vi "FipsAdjacent.vi"() -> (11 "Fips":i32[](array[numeric]))   [LabVIEW 2017] (continued)
County, SC\"\t45075\n\"Edgefield County, SC\"\t45037\t\"Columbia County, GA\"\t13073\n\"Edgefield County, SC\"\t45037\t\"Richmond County, GA\"\t13245\n\"Edgefield County, SC\"\t45037\t\"Aiken County, SC\"\t45003\n\"Edgefield County, SC\"\t45037\t\"Edgefield County, SC\"\t45037\n\"Edgefield County, SC\"\t45037\t\"Greenwood County, SC\"\t45047\n\"Edgefield County, SC\"\t45037\t\"McCormick County, SC\"\t45065\n\"Edgefield County, SC\"\t45037\t\"Saluda County, SC\"\t45081\n\"Fairfield County, SC\"\t45039\t\"Chester County, SC\"\t45023\n\"Fairfield County, SC\"\t45039\t\"Fairfield County, SC\"\t45039\n\"Fairfield County, SC\"\t45039\t\"Kershaw County, SC\"\t45055\n\"Fairfield County, SC\"\t45039\t\"Lancaster County, SC\"\t45057\n\"Fairfield County, SC\"\t45039\t\"Newberry County, SC\"\t45071\n\"Fairfield County, SC\"\t45039\t\"Richland County, SC\"\t45079\n\"Fairfield County, SC\"\t45039\t\"Union County, SC\"\t45087\n\"Florence County, SC\"\t45041\t\"Clarendon County, SC\"\t45027\n\"Florence County, SC\"\t45041\t\"Darlington County, SC\"\t45031\n\"Florence County, SC\"\t45041\t\"Dillon County, SC\"\t45033\n\"Florence County, SC\"\t45041\t\"Florence County, SC\"\t45041\n\"Florence County, SC\"\t45041\t\"Lee County, SC\"\t45061\n\"Florence County, SC\"\t45041\t\"Marion County, SC\"\t45067\n\"Florence County, SC\"\t45041\t\"Marlboro County, SC\"\t45069\n\"Florence County, SC\"\t45041\t\"Sumter County, SC\"\t45085\n\"Florence County, SC\"\t45041\t\"Williamsburg County, SC\"\t45089\n\"Georgetown County, SC\"\t45043\t\"Berkeley County, SC\"\t45015\n\"Georgetown County, SC\"\t45043\t\"Charleston County, SC\"\t45019\n\"Georgetown County, SC\"\t45043\t\"Georgetown County, SC\"\t45043\n\"Georgetown County, SC\"\t45043\t\"Horry County, SC\"\t45051\n\"Georgetown County, SC\"\t45043\t\"Marion County, SC\"\t45067\n\"Georgetown County, SC\"\t45043\t\"Williamsburg County, SC\"\t45089\n\"Greenville County, SC\"\t45045\t\"Henderson County, NC\"\t37089\n\"Greenville County, SC\"\t45045\t\"Polk County, NC\"\t37149\n\"Greenville County, SC\"\t45045\t\"Transylvania County, NC\"\t37175\n\"Greenville County, SC\"\t45045\t\"Abbeville County, SC\"\t45001\n\"Greenville County, SC\"\t45045\t\"Anderson County, SC\"\t45007\n\"Greenville County, SC\"\t45045\t\"Greenville County, SC\"\t45045\n\"Greenville County, SC\"\t45045\t\"Laurens County, SC\"\t45059\n\"Greenville County, SC\"\t45045\t\"Pickens County, SC\"\t45077\n\"Greenville County, SC\"\t45045\t\"Spartanburg County, SC\"\t45083\n\"Greenwood County, SC\"\t45047\t\"Abbeville County, SC\"\t45001\n\"Greenwood County, SC\"\t45047\t\"Edgefield County, SC\"\t45037\n\"Greenwood County, SC\"\t45047\t\"Greenwood County, SC\"\t45047\n\"Greenwood County, SC\"\t45047\t\"Laurens County, SC\"\t45059\n\"Greenwood County, SC\"\t45047\t\"McCormick County, SC\"\t45065\n\"Greenwood County, SC\"\t45047\t\"Newberry County, SC\"\t45071\n\"Greenwood County, SC\"\t45047\t\"Saluda County, SC\"\t45081\n\"Hampton County, SC\"\t45049\t\"Effingham County, GA\"\t13103\n\"Hampton County, SC\"\t45049\t\"Screven County, GA\"\t13251\n\"Hampton County, SC\"\t45049\t\"Allendale County, SC\"\t45005\n\"Hampton County, SC\"\t45049\t\"Bamberg County, SC\"\t45009\n\"Hampton County, SC\"\t45049\t\"Beaufort County, SC\"\t45013\n\"Hampton County, SC\"\t45049\t\"Colleton County, SC\"\t45029\n\"Hampton County, SC\"\t45049\t\"Hampton County, SC\"\t45049\n\"Hampton County, SC\"\t45049\t\"Jasper County, SC\"\t45053\n\"Horry County, SC\"\t45051\t\"Brunswick County, NC\"\t37019\n\"Horry County, SC\"\t45051\t\"Columbus County, NC\"\t37047\n\"Horry County, SC\"\t45051\t\"Robeson County, NC\"\t37155\n\"Horry County, SC\"\t45051\t\"Dillon County, SC\"\t45033\n\"Horry County, SC\"\t45051\t\"Georgetown County, SC\"\t45043\n\"Horry County, SC\"\t45051\t\"Horry County, SC\"\t45051\n\"Horry County, SC\"\t45051\t\"Marion County, SC\"\t45067\n\"Jasper County, SC\"\t45053\t\"Chatham County, GA\"\t13051\n\"Jasper County, SC\"\t45053\t\"Effingham County, GA\"\t13103\n\"Jasper County, SC\"\t45053\t\"Beaufort County, SC\"\t45013\n\"Jasper County, SC\"\t45053\t\"Hampton County, SC\"\t45049\n\"Jasper County, SC\"\t45053\t\"Jasper County, SC\"\t45053\n\"Kershaw County, SC\"\t45055\t\"Chesterfield County, SC\"\t45025\n\"Kershaw County, SC\"\t45055\t\"Darlington County, SC\"\t45031\n\"Kershaw County, SC\"\t45055\t\"Fairfield County, SC\"\t45039\n\"Kershaw County, SC\"\t45055\t\"Kershaw County, SC\"\t45055\n\"Kershaw County, SC\"\t45055\t\"Lancaster County, SC\"\t45057\n\"Kershaw County, SC\"\t45055\t\"Lee County, SC\"\t45061\n\"Kershaw County, SC\"\t45055\t\"Richland County, SC\"\t45079\n\"Kershaw County, SC\"\t45055\t\"Sumter County, SC\"\t45085\n\"Lancaster County, SC\"\t45057\t\"Mecklenburg County, NC\"\t37119\n\"Lancaster County, SC\"\t45057\t\"Union County, NC\"\t37179\n\"Lancaster County, SC\"\t45057\t\"Chester County, SC\"\t45023\n\"Lancaster County, SC\"\t45057\t\"Chesterfield County, SC\"\t45025\n\"Lancaster County, SC\"\t45057\t\"Fairfield County, SC\"\t45039\n\"Lancaster County, SC\"\t45057\t\"Kershaw County, SC\"\t45055\n\"Lancaster County, SC\"\t45057\t\"Lancaster County, SC\"\t45057\n\"Lancaster County, SC\"\t45057\t\"York County, SC\"\t45091\n\"Laurens County, SC\"\t45059\t\"Abbeville County, SC\"\t45001\n\"Laurens County, SC\"\t45059\t\"Anderson County, SC\"\t45007\n\"Laurens County, SC\"\t45059\t\"Greenville County, SC\"\t45045\n\"Laurens County, SC\"\t45059\t\"Greenwood County, SC\"\t45047\n\"Laurens County, SC\"\t45059\t\"Laurens County, SC\"\t45059\n\"Laurens County, SC\"\t45059\t\"Newberry County, SC\"\t45071\n\"Laurens County, SC\"\t45059\t\"Spartanburg County, SC\"\t45083\n\"Laurens County, SC\"\t45059\t\"Union County, SC\"\t45087\n\"Lee County, SC\"\t45061\t\"Darlington County, SC\"\t45031\n\"Lee County, SC\"\t45061\t\"Florence County, SC\"\t45041\n\"Lee County, SC\"\t45061\t\"Kershaw County, SC\"\t45055\n\"Lee County, SC\"\t45061\t\"Lee County, SC\"\t45061\n\"Lee County, SC\"\t45061\t\"Sumter County, SC\"\t45085\n\"Lexington County, SC\"\t45063\t\"Aiken County, SC\"\t45003\n\"Lexington County, SC\"\t45063\t\"Calhoun County, SC\"\t45017\n\"Lexington County, SC\"\t45063\t\"Lexington County, SC\"\t45063\n\"Lexington County, SC\"\t45063\t\"Newberry County, SC\"\t45071\n\"Lexington County, SC\"\t45063\t\"Orangeburg County, SC\"\t45075\n\"Lexington County, SC\"\t45063\t\"Richland County, SC\"\t45079\n\"Lexington County, SC\"\t45063\t\"Saluda County, SC\"\t45081\n\"McCormick County, SC\"\t45065\t\"Columbia County, GA\"\t13073\n\"McCormick County, SC\"\t45065\t\"Elbert County, GA\"\t13105\n\"McCormick County, SC\"\t45065\t\"Lincoln County, GA\"\t13181\n\"McCormick County, SC\"\t45065\t\"Abbeville County, SC\"\t45001\n\"McCormick County, SC\"\t45065\t\"Edgefield County, SC\"\t45037\n\"McCormick County, SC\"\t45065\t\"Greenwood County, SC\"\t45047\n\"McCormick County, SC\"\t45065\t\"McCormick County, SC\"\t45065\n\"Marion County, SC\"\t45067\t\"Dillon County, SC\"\t45033\n\"Marion County, SC\"\t45067\t\"Florence County, SC\"\t45041\n\"Marion County, SC\"\t45067\t\"Georgetown County, SC\"\t45043\n\"Marion County, SC\"\t45067\t\"Horry County, SC\"\t45051\n\"Marion County, SC\"\t45067\t\"Marion County, SC\"\t45067\n\"Marion County, SC\"\t45067\t\"Williamsburg County, SC\"\t45089\n\"Marlboro County, SC\"\t45069\t\"Anson County, NC\"\t37007\n\"Marlboro County, SC\"\t45069\t\"Richmond County, NC\"\t37153\n\"Marlboro County, SC\"\t45069\t\"Robeson County, NC\"\t37155\n\"Marlboro County, SC\"\t45069\t\"Scotland County, NC\"\t37165\n\"Marlboro County, SC\"\t45069\t\"Chesterfield County, SC\"\t45025\n\"Marlboro County, SC\"\t45069\t\"Darlington County, SC\"\t45031\n\"Marlboro County, SC\"\t45069\t\"Dillon County, SC\"\t45033\n\"Marlboro County, SC\"\t45069\t\"Florence County, SC\"\t45041\n\"Marlboro County, SC\"\t45069\t\"Marlboro County, SC\"\t45069\n\"Newberry County, SC\"\t45071\t\"Fairfield County, SC\"\t45039\n\"Newberry County, SC\"\t45071\t\"Greenwood County, SC\"\t45047\n\"Newberry County, SC\"\t45071\t\"Laurens County, SC\"\t45059\n\"Newberry County, SC\"\t45071\t\"Lexington County, SC\"\t45063\n\"Newberry County, SC\"\t45071\t\"Newberry County, SC\"\t45071\n\"Newberry County, SC\"\t45071\t\"Richland County, SC\"\t45079\n\"Newberry County, SC\"\t45071\t\"Saluda County, SC\"\t45081\n\"Newberry County, SC\"\t45071\t\"Union County, SC\"\t45087\n\"Oconee County, SC\"\t45073\t\"Franklin County, GA\"\t13119\n\"Oconee County, SC\"\t45073\t\"Habersham County, GA\"\t13137\n\"Oconee County, SC\"\t45073\t\"Hart County, GA\"\t13147\n\"Oconee County, SC\"\t45073\t\"Rabun County, GA\"\t13241\n\"Oconee County, SC\"\t45073\t\"Stephens County, GA\"\t13257\n\"Oconee County, SC\"\t45073\t\"Jackson County, NC\"\t37099\n\"Oconee County, SC\"\t45073\t\"Macon County, NC\"\t37113\n\"Oconee County, SC\"\t45073\t\"Transylvania County, NC\"\t37175\n\"Oconee County, SC\"\t45073\t\"Anderson County, SC\"\t45007\n\"Oconee County, SC\"\t45073\t\"Oconee County, SC\"\t45073\n\"Oconee County, SC\"\t45073\t\"Pickens County, SC\"\t45077\n\"Orangeburg County, SC\"\t45075\t\"Aiken County, SC\"\t45003\n\"Orangeburg County, SC\"\t45075\t\"Bamberg County, SC\"\t45009\n\"Orangeburg County, SC\"\t45075\t\"Barnwell County, SC\"\t45011\n\"Orangeburg County, SC\"\t45075\t\"Berkeley County, SC\"\t45015\n\"Orangeburg County, SC\"\t45075\t\"Calhoun County, SC\"\t45017\n\"Orangeburg County, SC\"\t45075\t\"Clarendon County, SC\"\t45027\n\"Orangeburg County, SC\"\t45075\t\"Colleton County, SC\"\t45029\n\"Orangeburg County, SC\"\t45075\t\"Dorchester County, SC\"\t45035\n\"Orangeburg County, SC\"\t45075\t\"Lexington County, SC\"\t45063\n\"Orangeburg County, SC\"\t45075\t\"Orangeburg County, SC\"\t45075\n\"Pickens County, SC\"\t45077\t\"Transylvania County, NC\"\t37175\n\"Pickens County, SC\"\t45077\t\"Anderson County, SC\"\t45007\n\"Pickens County, SC\"\t45077\t\"Greenville County, SC\"\t45045\n\"Pickens County, SC\"\t45077\t\"Oconee County, SC\"\t45073\n\"Pickens County, SC\"\t45077\t\"Pickens County, SC\"\t45077\n\"Richland County, SC\"\t45079\t\"Calhoun County, SC\"\t45017\n\"Richland County, SC\"\t45079\t\"Fairfield County, SC\"\t45039\n\"Richland County, SC\"\t45079\t\"Kershaw County, SC\"\t45055\n\"Richland County, SC\"\t45079\t\"Lexington County, SC\"\t45063\n\"Richland County, SC\"\t45079\t\"Newberry County, SC\"\t45071\n\"Richland County, SC\"\t45079\t\"Richland County, SC\"\t45079\n\"Richland County, SC\"\t45079\t\"Sumter County, SC\"\t45085\n\"Saluda County, SC\"\t45081\t\"Aiken County, SC\"\t45003\n\"Saluda County, SC\"\t45081\t\"Edgefield County, SC\"\t45037\n\"Saluda County, SC\"\t45081\t\"Greenwood County, SC\"\t45047\n\"Saluda County, SC\"\t45081\t\"Lexington County, SC\"\t45063\n\"Saluda County, SC\"\t45081\t\"Newberry County, SC\"\t45071\n\"Saluda County, SC\"\t45081\t\"Saluda County, SC\"\t45081\n\"Spartanburg County, SC\"\t45083\t\"Polk County, NC\"\t37149\n\"Spartanburg County, SC\"\t45083\t\"Rutherford County, NC\"\t37161\n\"Spartanburg County, SC\"\t45083\t\"Cherokee County, SC\"\t45021\n\"Spartanburg County, SC\"\t45083\t\"Greenville County, SC\"\t45045\n\"Spartanburg County, SC\"\t45083\t\"Laurens County, SC\"\t45059\n\"Spartanburg County, SC\"\t45083\t\"Spartanburg County, SC\"\t45083\n\"Spartanburg County, SC\"\t45083\t\"Union County, SC\"\t45087\n\"Sumter County, SC\"\t45085\t\"Calhoun County, SC\"\t45017\n\"Sumter County, SC\"\t45085\t\"Clarendon County, SC\"\t45027\n\"Sumter County, SC\"\t45085\t\"Florence County, SC\"\t45041\n\"Sumter County, SC\"\t45085\t\"Kershaw County, SC\"\t45055\n\"Sumter County, SC\"\t45085\t\"Lee County, SC\"\t45061\n\"Sumter County, SC\"\t45085\t\"Richland County, SC\"\t45079\n\"Sumter County, SC\"\t45085\t\"Sumter County, SC\"\t45085\n\"Union County, SC\"\t45087\t\"Cherokee County, SC\"\t45021\n\"Union County, SC\"\t45087\t\"Chester County, SC\"\t45023\n\"Union County, SC\"\t45087\t\"Fairfield County, SC\"\t45039\n\"Union County, SC\"\t45087\t\"Laurens County, SC\"\t45059\n\"Union County, SC\"\t45087\t\"Newberry County, SC\"\t45071\n\"Union County, SC\"\t45087\t\"Spartanburg County, SC\"\t45083\n\"Union County, SC\"\t45087\t\"Union County, SC\"\t45087\n\"Union County, SC\"\t45087\t\"York County, SC\"\t45091\n\"Williamsburg County, SC\"\t45089\t\"Berkeley County, SC\"\t45015\n\"Williamsburg County, SC\"\t45089\t\"Clarendon County, SC\"\t45027\n\"Williamsburg County, SC\"\t45089\t\"Florence County, SC\"\t45041\n\"Williamsburg County, SC\"\t45089\t\"Georgetown County, SC\"\t45043\n\"Williamsburg County, SC\"\t45089\t\"Marion County, SC\"\t45067\n\"Williamsburg County, SC\"\t45089\t\"Williamsburg County, SC\"\t45089\n\"York County, SC\"\t45091\t\"Cleveland County, NC\"\t37045\n\"York County, SC\"\t45091\t\"Gaston County, NC\"\t37071\n\"York County, SC\"\t45091\t\"Mecklenburg County, NC\"\t37119\n\"York County, SC\"\t45091\t\"Cherokee County, SC\"\t45021\n\"York County, SC\"\t45091\t\"Chester County, SC\"\t45023\n\"York County, SC\"\t45091\t\"Lancaster County, SC\"\t45057\n\"York County, SC\"\t45091\t\"Union County, SC\"\t45087\n\"York County, SC\"\t45091\t\"York County, SC\"\t45091\n\"Aurora County, SD\"\t46003\t\"Aurora County, SD\"\t46003\n\"Aurora County, SD\"\t46003\t\"Brule County, SD\"\t46015\n\"Aurora County, SD\"\t46003\t\"Charles Mix County, SD\"\t46023\n\"Aurora County, SD\"\t46003\t\"Davison County, SD\"\t46035\n\"Aurora County, SD\"\t46003\t\"Douglas County, SD\"\t46043\n\"Aurora County, SD\"\t46003\t\"Jerauld County, SD\"\t46073\n\"Aurora County, SD\"\t46003\t\"Sanborn County, SD\"\t46111\n\"Beadle County, SD\"\t46005\t\"Beadle County, SD\"\t46005\n\"Beadle County, SD\"\t46005\t\"Clark County, SD\"\t46025\n\"Beadle County, SD\"\t46005\t\"Hand County, SD\"\t46059\n\"Beadle County, SD\"\t46005\t\"Jerauld County, SD\"\t46073\n\"Beadle County, SD\"\t46005\t\"Kingsbury County, SD\"\t46077\n\"Beadle County, SD\"\t46005\t\"Sanborn County, SD\"\t46111\n\"Beadle County, SD\"\t46005\t\"Spink County, SD\"\t46115\n\"Bennett County, SD\"\t46007\t\"Cherry County, NE\"\t31031\n\"Bennett County, SD\"\t46007\t\"Bennett County, SD\"\t46007\n\"Bennett County, SD\"\t46007\t\"Jackson County, SD\"\t46071\n\"Bennett County, SD\"\t46007\t\"Mellette County, SD\"\t46095\n\"Bennett County, SD\"\t46007\t\"Shannon County, SD\"\t46113\n\"Bennett County, SD\"\t46007\t\"Todd County, SD\"\t46121\n\"Bon Homme County, SD\"\t46009\t\"Knox County, NE\"\t31107\n\"Bon Homme County, SD\"\t46009\t\"Bon Homme County, SD\"\t46009\n\"Bon Homme County, SD\"\t46009\t\"Charles Mix County, SD\"\t46023\n\"Bon Homme County, SD\"\t46009\t\"Hutchinson County, SD\"\t46067\n\"Bon Homme County, SD\"\t46009\t\"Yankton County, SD\"\t46135\n\"Brookings County, SD\"\t46011\t\"Lincoln County, MN\"\t27081\n\"Brookings County, SD\"\t46011\t\"Pipestone County, MN\"\t27117\n\"Brookings County, SD\"\t46011\t\"Brookings County, SD\"\t46011\n\"Brookings County, SD\"\t46011\t\"Deuel County, SD\"\t46039\n\"Brookings County, SD\"\t46011\t\"Hamlin County, SD\"\t46057\n\"Brookings County, SD\"\t46011\t\"Kingsbury County, SD\"\t46077\n\"Brookings County, SD\"\t46011\t\"Lake County, SD\"\t46079\n\"Brookings County, SD\"\t46011\t\"Moody County, SD\"\t46101\n\"Brown County, SD\"\t46013\t\"Dickey County, ND\"\t38021\n\"Brown County, SD\"\t46013\t\"Sargent County, ND\"\t38081\n\"Brown County, SD\"\t46013\t\"Brown County, SD\"\t46013\n\"Brown County, SD\"\t46013\t\"Day County, SD\"\t46037\n\"Brown County, SD\"\t46013\t\"Edmunds County, SD\"\t46045\n\"Brown County, SD\"\t46013\t\"Faulk County, SD\"\t46049\n\"Brown County, SD\"\t46013\t\"McPherson County, SD\"\t46089\n\"Brown County, SD\"\t46013\t\"Marshall County, SD\"\t46091\n\"Brown County, SD\"\t46013\t\"Spink County, SD\"\t46115\n\"Brule County, SD\"\t46015\t\"Aurora County, SD\"\t46003\n\"Brule County, SD\"\t46015\t\"Brule County, SD\"\t46015\n\"Brule County, SD\"\t46015\t\"Buffalo County, SD\"\t46017\n\"Brule County, SD\"\t46015\t\"Charles Mix County, SD\"\t46023\n\"Brule County, SD\"\t46015\t\"Jerauld County, SD\"\t46073\n\"Brule County, SD\"\t46015\t\"Lyman County, SD\"\t46085\n\"Buffalo County, SD\"\t46017\t\"Brule County, SD\"\t46015\n\"Buffalo County, SD\"\t46017\t\"Buffalo County, SD\"\t46017\n\"Buffalo County, SD\"\t46017\t\"Hand County, SD\"\t46059\n\"Buffalo County, SD\"\t46017\t\"Hyde County, SD\"\t46069\n\"Buffalo County, SD\"\t46017\t\"Jerauld County, SD\"\t46073\n\"Buffalo County, SD\"\t46017\t\"Lyman County, SD\"\t46085\n\"Butte County, SD\"\t46019\t\"Carter County, MT\"\t30011\n\"Butte County, SD\"\t46019\t\"Butte County, SD\"\t46019\n\"Butte County, SD\"\t46019\t\"Harding County, SD\"\t46063\n\"Butte County, SD\"\t46019\t\"Lawrence County, SD\"\t46081\n\"Butte County, SD\"\t46019\t\"Meade County, SD\"\t46093\n\"Butte County, SD\"\t46019\t\"Perkins County, SD\"\t46105\n\"Butte County, SD\"\t46019\t\"Crook County, WY\"\t56011\n\"Campbell County, SD\"\t46021\t\"Emmons County, ND\"\t38029\n\"Campbell County, SD\"\t46021\t\"McIntosh County, ND\"\t38051\n\"Campbell County, SD\"\t46021\t\"Campbell County, SD\"\t46021\n\"Campbell County, SD\"\t46021\t\"Corson County, SD\"\t46031\n\"Campbell County, SD\"\t46021\t\"McPherson County, SD\"\t46089\n\"Campbell County, SD\"\t46021\t\"Walworth County, SD\"\t46129\n\"Charles Mix County, SD\"\t46023\t\"Boyd County, NE\"\t31015\n\"Charles Mix County, SD\"\t46023\t\"Knox County, NE\"\t31107\n\"Charles Mix County, SD\"\t46023\t\"Aurora County, SD\"\t46003\n\"Charles Mix County, SD\"\t46023\t\"Bon Homme County, SD\"\t46009\n\"Charles Mix County, SD\"\t46023\t\"Brule County, SD\"\t46015\n\"Charles Mix County, SD\"\t46023\t\"Charles Mix County, SD\"\t46023\n\"Charles Mix County, SD\"\t46023\t\"Douglas County, SD\"\t46043\n\"Charles Mix County, SD\"\t46023\t\"Gregory County, SD\"\t46053\n\"Charles Mix County, SD\"\t46023\t\"Hutchinson County, SD\"\t46067\n\"Charles Mix County, SD\"\t46023\t\"Lyman County, SD\"\t46085\n\"Clark County, SD\"\t46025\t\"Beadle County, SD\"\t46005\n\"Clark County, SD\"\t46025\t\"Clark County, SD\"\t46025\n\"Clark County, SD\"\t46025\t\"Codington County, SD\"\t46029\n\"Clark County, SD\"\t46025\t\"Day County, SD\"\t46037\n\"Clark County, SD\"\t46025\t\"Hamlin County, SD\"\t46057\n\"Clark County, SD\"\t46025\t\"Kingsbury County, SD\"\t46077\n\"Clark County, SD\"\t46025\t\"Spink County, SD\"\t46115\n\"Clay County, SD\"\t46027\t\"Cedar County, NE\"\t31027\n\"Clay County, SD\"\t46027\t\"Dixon County, NE\"\t31051\n\"Clay County, SD\"\t46027\t\"Clay County, SD\"\t46027\n\"Clay County, SD\"\t46027\t\"Lincoln County, SD\"\t46083\n\"Clay County, SD\"\t46027\t\"Turner County, SD\"\t46125\n\"Clay County, SD\"\t46027\t\"Union County, SD\"\t46127\n\"Clay County, SD\"\t46027\t\"Yankton County, SD\"\t46135\n\"Codington County, SD\"\t46029\t\"Clark County, SD\"\t46025\n\"Codington County, SD\"\t46029\t\"Codington County, SD\"\t46029\n\"Codington County, SD\"\t46029\t\"Day County, SD\"\t46037\n\"Codington County, SD\"\t46029\t\"Deuel County, SD\"\t46039\n\"Codington County, SD\"\t46029\t\"Grant County, SD\"\t46051\n\"Codington County, SD\"\t46029\t\"Hamlin County, SD\"\t46057\n\"Corson County, SD\"\t46031\t\"Adams County, ND\"\t38001\n\"Corson County, SD\"\t46031\t\"Emmons County, ND\"\t38029\n\"Corson County, SD\"\t46031\t\"Sioux County, ND\"\t38085\n\"Corson County, SD\"\t46031\t\"Campbell County, SD\"\t46021\n\"Corson County, SD\"\t46031\t\"Corson County, SD\"\t46031\n\"Corson County, SD\"\t46031\t\"Dewey County, SD\"\t46041\n\"Corson County, SD\"\t46031\t\"Perkins County, SD\"\t46105\n\"Corson County, SD\"\t46031\t\"Walworth County, SD\"\t46129\n\"Corson County, SD\"\t46031\t\"Ziebach County, SD\"\t46137\n\"Custer County, SD\"\t46033\t\"Custer County, SD\"\t46033\n\"Custer County, SD\"\t46033\t\"Fall River County, SD\"\t46047\n\"Custer County, SD\"\t46033\t\"Pennington County, SD\"\t46103\n\"Custer County, SD\"\t46033\t\"Shannon County, SD\"\t46113\n\"Custer County, SD\"\t46033\t\"Niobrara County, WY\"\t56027\n\"Custer County, SD\"\t46033\t\"Weston County, WY\"\t56045\n\"Davison County, SD\"\t46035\t\"Aurora County, SD\"\t46003\n\"Davison County, SD\"\t46035\t\"Davison County, SD\"\t46035\n\"Davison County, SD\"\t46035\t\"Douglas County, SD\"\t46043\n\"Davison County, SD\"\t46035\t\"Hanson County, SD\"\t46061\n\"Davison County, SD\"\t46035\t\"Hutchinson County, SD\"\t46067\n\"Davison County, SD\"\t46035\t\"Sanborn County, SD\"\t46111\n\"Day County, SD\"\t46037\t\"Brown County, SD\"\t46013\n\"Day County, SD\"\t46037\t\"Clark County, SD\"\t46025\n\"Day County, SD\"\t46037\t\"Codington County, SD\"\t46029\n\"Day County, SD\"\t46037\t\"Day County, SD\"\t46037\n\"Day County, SD\"\t46037\t\"Grant County, SD\"\t46051\n\"Day County, SD\"\t46037\t\"Marshall County, SD\"\t46091\n\"Day County, SD\"\t46037\t\"Roberts County, SD\"\t46109\n\"Day County, SD\"\t46037\t\"Spink County, SD\"\t46115\n\"Deuel County, SD\"\t46039\t\"Lac qui Parle County, MN\"\t27073\n\"Deuel County, SD\"\t46039\t\"Lincoln County, MN\"\t27081\n\"Deuel County, SD\"\t46039\t\"Yellow Medicine County, MN\"\t27173\n\"Deuel County, SD\"\t46039\t\"Brookings County, SD\"\t46011\n\"Deuel County, SD\"\t46039\t\"Codington County, SD\"\t46029\n\"Deuel County, SD\"\t46039\t\"Deuel County, SD\"\t46039\n\"Deuel County, SD\"\t46039\t\"Grant County, SD\"\t46051\n\"Deuel County, SD\"\t46039\t\"Hamlin County, SD\"\t46057\n\"Dewey County, SD\"\t46041\t\"Corson County, SD\"\t46031\n\"Dewey County, SD\"\t46041\t\"Dewey County, SD\"\t46041\n\"Dewey County, SD\"\t46041\t\"Haakon County, SD\"\t46055\n\"Dewey County, SD\"\t46041\t\"Potter County, SD\"\t46107\n\"Dewey County, SD\"\t46041\t\"Stanley County, SD\"\t46117\n\"Dewey County, SD\"\t46041\t\"Sully County, SD\"\t46119\n\"Dewey County, SD\"\t46041\t\"Walworth County, SD\"\t46129\n\"Dewey County, SD\"\t46041\t\"Ziebach County, SD\"\t46137\n\"Douglas County, SD\"\t46043\t\"Aurora County, SD\"\t46003\n\"Douglas County, SD\"\t46043\t\"Charles Mix County, SD\"\t46023\n\"Douglas County, SD\"\t46043\t\"Davison County, SD\"\t46035\n\"Douglas County, SD\"\t46043\t\"Douglas County, SD\"\t46043\n\"Douglas County, SD\"\t46043\t\"Hutchinson County, SD\"\t46067\n\"Edmunds County, SD\"\t46045\t\"Brown County, SD\"\t46013\n\"Edmunds County, SD\"\t46045\t\"Edmunds County, SD\"\t46045\n\"Edmunds County, SD\"\t46045\t\"Faulk County, SD\"\t46049\n\"Edmunds County, SD\"\t46045\t\"McPherson County, SD\"\t46089\n\"Edmunds County, SD\"\t46045\t\"Potter County, SD\"\t46107\n\"Edmunds County, SD\"\t46045\t\"Walworth County, SD\"\t46129\n\"Fall River County, SD\"\t46047\t\"Dawes County, NE\"\t31045\n\"Fall River County, SD\"\t46047\t\"Sioux County, NE\"\t31165\n\"Fall River County, SD\"\t46047\t\"Custer County, SD\"\t46033\n\"Fall River County, SD\"\t46047\t\"Fall River County, SD\"\t46047\n\"Fall River County, SD\"\t46047\t\"Shannon County, SD\"\t46113\n\"Fall River County, SD\"\t46047\t\"Niobrara County, WY\"\t56027\n\"Faulk County, SD\"\t46049\t\"Brown County, SD\"\t46013\n\"Faulk County, SD\"\t46049\t\"Edmunds County, SD\"\t46045\n\"Faulk County, SD\"\t46049\t\"Faulk County, SD\"\t46049\n\"Faulk County, SD\"\t46049\t\"Hand County, SD\"\t46059\n\"Faulk County, SD\"\t46049\t\"Hyde County, SD\"\t46069\n\"Faulk County, SD\"\t46049\t\"Potter County, SD\"\t46107\n\"Faulk County, SD\"\t46049\t\"Spink County, SD\"\t46115\n\"Grant County, SD\"\t46051\t\"Big Stone County, MN\"\t27011\n\"Grant County, SD\"\t46051\t\"Lac qui Parle County, MN\"\t27073\n\"Grant County, SD\"\t46051\t\"Codington County, SD\"\t46029\n\"Grant County, SD\"\t46051\t\"Day County, SD\"\t46037\n\"Grant County, SD\"\t46051\t\"Deuel County, SD\"\t46039\n\"Grant County, SD\"\t46051\t\"Grant County, SD\"\t46051\n\"Grant County, SD\"\t46051\t\"Roberts County, SD\"\t46109\n\"Gregory County, SD\"\t46053\t\"Boyd County, NE\"\t31015\n\"Gregory County, SD\"\t46053\t\"Keya Paha County, NE\"\t31103\n\"Gregory County, SD\"\t46053\t\"Charles Mix County, SD\"\t46023\n\"Gregory County, SD\"\t46053\t\"Gregory County, SD\"\t46053\n\"Gregory County, SD\"\t46053\t\"Lyman County, SD\"\t46085\n\"Gregory County, SD\"\t46053\t\"Tripp County, SD\"\t46123\n\"Haakon County, SD\"\t46055\t\"Dewey County, SD\"\t46041\n\"Haakon County, SD\"\t46055\t\"Haakon County, SD\"\t46055\n\"Haakon County, SD\"\t46055\t\"Jackson County, SD\"\t46071\n\"Haakon County, SD\"\t46055\t\"Jones County, SD\"\t46075\n\"Haakon County, SD\"\t46055\t\"Meade County, SD\"\t46093\n\"Haakon County, SD\"\t46055\t\"Pennington County, SD\"\t46103\n\"Haakon County, SD\"\t46055\t\"Stanley County, SD\"\t46117\n\"Haakon County, SD\"\t46055\t\"Ziebach County, SD\"\t46137\n\"Hamlin County, SD\"\t46057\t\"Brookings County, SD\"\t46011\n\"Hamlin County, SD\"\t46057\t\"Clark County, SD\"\t46025\n\"Hamlin County, SD\"\t46057\t\"Codington County, SD\"\t46029\n\"Hamlin County, SD\"\t46057\t\"Deuel County, SD\"\t46039\n\"Hamlin County, SD\"\t46057\t\"Hamlin County, SD\"\t46057\n\"Hamlin County, SD\"\t46057\t\"Kingsbury County, SD\"\t46077\n\"Hand County, SD\"\t46059\t\"Beadle County, SD\"\t46005\n\"Hand County, SD\"\t46059\t\"Buffalo County, SD\"\t46017\n\"Hand County, SD\"\t46059\t\"Faulk County, SD\"\t46049\n\"Hand County, SD\"\t46059\t\"Hand County, SD\"\t46059\n\"Hand County, SD\"\t46059\t\"Hyde County, SD\"\t46069\n\"Hand County, SD\"\t46059\t\"Jerauld County, SD\"\t46073\n\"Hand County, SD\"\t46059\t\"Spink County, SD\"\t46115\n\"Hanson County, SD\"\t46061\t\"Davison County, SD\"\t46035\n\"Hanson County, SD\"\t46061\t\"Hanson County, SD\"\t46061\n\"Hanson County, SD\"\t46061\t\"Hutchinson County, SD\"\t46067\n\"Hanson County, SD\"\t46061\t\"McCook County, SD\"\t46087\n\"Hanson County, SD\"\t46061\t\"Miner County, SD\"\t46097\n\"Hanson County, SD\"\t46061\t\"Sanborn County, SD\"\t46111\n\"Harding County, SD\"\t46063\t\"Carter County, MT\"\t30011\n\"Harding County, SD\"\t46063\t\"Fallon County, MT\"\t30025\n\"Harding County, SD\"\t46063\t\"Adams County, ND\"\t38001\n\"Harding County, SD\"\t46063\t\"Bowman County, ND\"\t38011\n\"Harding County, SD\"\t46063\t\"Butte County, SD\"\t46019\n\"Harding County, SD\"\t46063\t\"Harding County, SD\"\t46063\n\"Harding County, SD\"\t46063\t\"Perkins County, SD\"\t46105\n\"Hughes County, SD\"\t46065\t\"Hughes County, SD\"\t46065\n\"Hughes County, SD\"\t46065\t\"Hyde County, SD\"\t46069\n\"Hughes County, SD\"\t46065\t\"Lyman County, SD\"\t46085\n\"Hughes County, SD\"\t46065\t\"Stanley County, SD\"\t46117\n\"Hughes County, SD\"\t46065\t\"Sully County, SD\"\t46119\n\"Hutchinson County, SD\"\t46067\t\"Bon Homme County, SD\"\t46009\n\"Hutchinson County, SD\"\t46067\t\"Charles Mix County, SD\"\t46023\n\"Hutchinson County, SD\"\t46067\t\"Davison County, SD\"\t46035\n\"Hutchinson County, SD\"\t46067\t\"Douglas County, SD\"\t46043\n\"Hutchinson County, SD\"\t46067\t\"Hanson County, SD\"\t46061\n\"Hutchinson County, SD\"\t46067\t\"Hutchinson County, SD\"\t46067\n\"Hutchinson County, SD\"\t46067\t\"McCook County, SD\"\t46087\n\"Hutchinson County, SD\"\t46067\t\"Turner County, SD\"\t46125\n\"Hutchinson County, SD\"\t46067\t\"Yankton County, SD\"\t46135\n\"Hyde County, SD\"\t46069\t\"Buffalo County, SD\"\t46017\n\"Hyde County, SD\"\t46069\t\"Faulk County, SD\"\t46049\n\"Hyde County, SD\"\t46069\t\"Hand County, SD\"\t46059\n\"Hyde County, SD\"\t46069\t\"Hughes County, SD\"\t46065\n\"Hyde County, SD\"\t46069\t\"Hyde County, SD\"\t46069\n\"Hyde County, SD\"\t46069\t\"Lyman County, SD\"\t46085\n\"Hyde County, SD\"\t46069\t\"Potter County, SD\"\t46107\n\"Hyde County, SD\"\t46069\t\"Sully County, SD\"\t46119\n\"Jackson County, SD\"\t46071\t\"Bennett County, SD\"\t46007\n\"Jackson County, SD\"\t46071\t\"Haakon County, SD\"\t46055\n\"Jackson County, SD\"\t46071\t\"Jackson County, SD\"\t46071\n\"Jackson County, SD\"\t46071\t\"Jones County, SD\"\t46075\n\"Jackson County, SD\"\t46071\t\"Mellette County, SD\"\t46095\n\"Jackson County, SD\"\t46071\t\"Pennington County, SD\"\t46103\n\"Jackson County, SD\"\t46071\t\"Shannon County, SD\"\t46113\n\"Jackson County, SD\"\t46071\t\"Todd County, SD\"\t46121\n\"Jerauld County, SD\"\t46073\t\"Aurora County, SD\"\t46003\n\"Jerauld County, SD\"\t46073\t\"Beadle County, SD\"\t46005\n\"Jerauld County, SD\"\t46073\t\"Brule County, SD\"\t46015\n\"Jerauld County, SD\"\t46073\t\"Buffalo County, SD\"\t46017\n\"Jerauld County, SD\"\t46073\t\"Hand County, SD\"\t46059\n\"Jerauld County, SD\"\t46073\t\"Jerauld County, SD\"\t46073\n\"Jerauld County, SD\"\t46073\t\"Sanborn County, SD\"\t46111\n\"Jones County, SD\"\t46075\t\"Haakon County, SD\"\t46055\n\"Jones County, SD\"\t46075\t\"Jackson County, SD\"\t46071\n\"Jones County, SD\"\t46075\t\"Jones County, SD\"\t46075\n\"Jones County, SD\"\t46075\t\"Lyman County, SD\"\t46085\n\"Jones County, SD\"\t46075\t\"Mellette County, SD\"\t46095\n\"Jones County, SD\"\t46075\t\"Stanley County, SD\"\t46117\n\"Kingsbury County, SD\"\t46077\t\"Beadle County, SD\"\t46005\n\"Kingsbury County, SD\"\t46077\t\"Brookings County, SD\"\t46011\n\"Kingsbury County, SD\"\t46077\t\"Clark County, SD\"\t46025\n\"Kingsbury County, SD\"\t46077\t\"Hamlin County, SD\"\t46057\n\"Kingsbury County, SD\"\t46077\t\"Kingsbury County, SD\"\t46077\n\"Kingsbury County, SD\"\t46077\t\"Lake County, SD\"\t46079\n\"Kingsbury County, SD\"\t46077\t\"Miner County, SD\"\t46097\n\"Kingsbury County, SD\"\t46077\t\"Sanborn County, SD\"\t46111\n\"Lake County, SD\"\t46079\t\"Brookings County, SD\"\t46011\n\"Lake County, SD\"\t46079\t\"Kingsbury County, SD\"\t46077\n\"Lake County, SD\"\t46079\t\"Lake County, SD\"\t46079\n\"Lake County, SD\"\t46079\t\"McCook County, SD\"\t46087\n\"Lake County, SD\"\t46079\t\"Miner County, SD\"\t46097\n\"Lake County, SD\"\t46079\t\"Minnehaha County, SD\"\t46099\n\"Lake County, SD\"\t46079\t\"Moody County, SD\"\t46101\n\"Lawrence County, SD\"\t46081\t\"Butte County, SD\"\t46019\n\"Lawrence County, SD\"\t46081\t\"Lawrence County, SD\"\t46081\n\"Lawrence County, SD\"\t46081\t\"Meade County, SD\"\t46093\n\"Lawrence County, SD\"\t46081\t\"Pennington County, SD\"\t46103\n\"Lawrence County, SD\"\t46081\t\"Crook County, WY\"\t56011\n\"Lawrence County, SD\"\t46081\t\"Weston County, WY\"\t56045\n\"Lincoln County, SD\"\t46083\t\"Lyon County, IA\"\t19119\n\"Lincoln County, SD\"\t46083\t\"Sioux County, IA\"\t19167\n\"Lincoln County, SD\"\t46083\t\"Clay County, SD\"\t46027\n\"Lincoln County, SD\"\t46083\t\"Lincoln County, SD\"\t46083\n\"Lincoln County, SD\"\t46083\t\"Minnehaha County, SD\"\t46099\n\"Lincoln County, SD\"\t46083\t\"Turner County, SD\"\t46125\n\"Lincoln County, SD\"\t46083\t\"Union County, SD\"\t46127\n\"Lyman County, SD\"\t46085\t\"Brule County, SD\"\t46015\n\"Lyman County, SD\"\t46085\t\"Buffalo County, SD\"\t46017\n\"Lyman County, SD\"\t46085\t\"Charles Mix County, SD\"\t46023\n\"Lyman County, SD\"\t46085\t\"Gregory County, SD\"\t46053\n\"Lyman County, SD\"\t46085\t\"Hughes County, SD\"\t46065\n\"Lyman County, SD\"\t46085\t\"Hyde County, SD\"\t46069\n\"Lyman County, SD\"\t46085\t\"Jones County, SD\"\t46075\n\"Lyman County, SD\"\t46085\t\"Lyman County, SD\"\t46085\n\"Lyman County, SD\"\t46085\t\"Mellette County, SD\"\t46095\n\"Lyman County, SD\"\t46085\t\"Stanley County, SD\"\t46117\n\"Lyman County, SD\"\t46085\t\"Tripp County, SD\"\t46123\n\"McCook County, SD\"\t46087\t\"Hanson County, SD\"\t46061\n\"McCook County, SD\"\t46087\t\"Hutchinson County, SD\"\t46067\n\"McCook County, SD\"\t46087\t\"Lake County, SD\"\t46079\n\"McCook County, SD\"\t46087\t\"McCook County, SD\"\t46087\n\"McCook County, SD\"\t46087\t\"Miner County, SD\"\t46097\n\"McCook County, SD\"\t46087\t\"Minnehaha County, SD\"\t46099\n\"McCook County, SD\"\t46087\t\"Turner County, SD\"\t46125\n\"McPherson County, SD\"\t46089\t\"Dickey County, ND\"\t38021\n\"McPherson County, SD\"\t46089\t\"McIntosh County, ND\"\t38051\n\"McPherson County, SD\"\t46089\t\"Brown County, SD\"\t46013\n\"McPherson County, SD\"\t46089\t\"Campbell County, SD\"\t46021\n\"McPherson County, SD\"\t46089\t\"Edmunds County, SD\"\t46045\n\"McPherson County, SD\"\t46089\t\"McPherson County, SD\"\t46089\n\"McPherson County, SD\"\t46089\t\"Walworth County, SD\"\t46129\n\"Marshall County, SD\"\t46091\t\"Richland County, ND\"\t38077\n\"Marshall County, SD\"\t46091\t\"Sargent County, ND\"\t38081\n\"Marshall County, SD\"\t46091\t\"Brown County, SD\"\t46013\n\"Marshall County, SD\"\t46091\t\"Day County, SD\"\t46037\n\"Marshall County, SD\"\t46091\t\"Marshall County, SD\"\t46091\n\"Marshall County, SD\"\t46091\t\"Roberts County, SD\"\t46109\n\"Meade County, SD\"\t46093\t\"Butte County, SD\"\t46019\n\"Meade County, SD\"\t46093\t\"Haakon County, SD\"\t46055\n\"Meade County, SD\"\t46093\t\"Lawrence County, SD\"\t46081\n\"Meade County, SD\"\t46093\t\"Meade County, SD\"\t46093\n\"Meade County, SD\"\t46093\t\"Pennington County, SD\"\t46103\n\"Meade County, SD\"\t46093\t\"Perkins County, SD\"\t46105\n\"Meade County, SD\"\t46093\t\"Ziebach County, SD\"\t46137\n\"Mellette County, SD\"\t46095\t\"Bennett County, SD\"\t46007\n\"Mellette County, SD\"\t46095\t\"Jackson County, SD\"\t46071\n\"Mellette County, SD\"\t46095\t\"Jones County, SD\"\t46075\n\"Mellette County, SD\"\t46095\t\"Lyman County, SD\"\t46085\n\"Mellette County, SD\"\t46095\t\"Mellette County, SD\"\t46095\n\"Mellette County, SD\"\t46095\t\"Todd County, SD\"\t46121\n\"Mellette County, SD\"\t46095\t\"Tripp County, SD\"\t46123\n\"Miner County, SD\"\t46097\t\"Hanson County, SD\"\t46061\n\"Miner County, SD\"\t46097\t\"Kingsbury County, SD\"\t46077\n\"Miner County, SD\"\t46097\t\"Lake County, SD\"\t46079\n\"Miner County, SD\"\t46097\t\"McCook County, SD\"\t46087\n\"Miner County, SD\"\t46097\t\"Miner County, SD\"\t46097\n\"Miner County, SD\"\t46097\t\"Sanborn County, SD\"\t46111\n\"Minnehaha County, SD\"\t46099\t\"Lyon County, IA\"\t19119\n\"Minnehaha County, SD\"\t46099\t\"Pipestone County, MN\"\t27117\n\"Minnehaha County, SD\"\t46099\t\"Rock County, MN\"\t27133\n\"Minnehaha County, SD\"\t46099\t\"Lake County, SD\"\t46079\n\"Minnehaha County, SD\"\t46099\t\"Lincoln County, SD\"\t46083\n\"Minnehaha County, SD\"\t46099\t\"McCook County, SD\"\t46087\n\"Minnehaha County, SD\"\t46099\t\"Minnehaha County, SD\"\t46099\n\"Minnehaha County, SD\"\t46099\t\"Moody County, SD\"\t46101\n\"Minnehaha County, SD\"\t46099\t\"Turner County, SD\"\t46125\n\"Moody County, SD\"\t46101\t\"Lincoln County, MN\"\t27081\n\"Moody County, SD\"\t46101\t\"Pipestone County, MN\"\t27117\n\"Moody County, SD\"\t46101\t\"Rock County, MN\"\t27133\n\"Moody County, SD\"\t46101\t\"Brookings County, SD\"\t46011\n\"Moody County, SD\"\t46101\t\"Lake County, SD\"\t46079\n\"Moody County, SD\"\t46101\t\"Minnehaha County, SD\"\t46099\n\"Moody County, SD\"\t46101\t\"Moody County, SD\"\t46101\n\"Pennington County, SD\"\t46103\t\"Custer County, SD\"\t46033\n\"Pennington County, SD\"\t46103\t\"Haakon County, SD\"\t46055\n\"Pennington County, SD\"\t46103\t\"Jackson County, SD\"\t46071\n\"Pennington County, SD\"\t46103\t\"Lawrence County, SD\"\t46081\n\"Pennington County, SD\"\t46103\t\"Meade County, SD\"\t46093\n\"Pennington County, SD\"\t46103\t\"Pennington County, SD\"\t46103\n\"Pennington County, SD\"\t46103\t\"Shannon County, SD\"\t46113\n\"Pennington County, SD\"\t46103\t\"Weston County, WY\"\t56045\n\"Perkins County, SD\"\t46105\t\"Adams County, ND\"\t38001\n\"Perkins County, SD\"\t46105\t\"Butte County, SD\"\t46019\n\"Perkins County, SD\"\t46105\t\"Corson County, SD\"\t46031\n\"Perkins County, SD\"\t46105\t\"Harding County, SD\"\t46063\n\"Perkins County, SD\"\t46105\t\"Meade County, SD\"\t46093\n\"Perkins County, SD\"\t46105\t\"Perkins County, SD\"\t46105\n\"Perkins County, SD\"\t46105\t\"Ziebach County, SD\"\t46137\n\"Potter County, SD\"\t46107\t\"Dewey County, SD\"\t46041\n\"Potter County, SD\"\t46107\t\"Edmunds County, SD\"\t46045\n\"Potter County, SD\"\t46107\t\"Faulk County, SD\"\t46049\n\"Potter County, SD\"\t46107\t\"Hyde County, SD\"\t46069\n\"Potter County, SD\"\t46107\t\"Potter County, SD\"\t46107\n\"Potter County, SD\"\t46107\t\"Sully County, SD\"\t46119\n\"Potter County, SD\"\t46107\t\"Walworth County, SD\"\t46129\n\"Roberts County, SD\"\t46109\t\"Big Stone County, MN\"\t27011\n\"Roberts County, SD\"\t46109\t\"Traverse County, MN\"\t27155\n\"Roberts County, SD\"\t46109\t\"Richland County, ND\"\t38077\n\"Roberts County, SD\"\t46109\t\"Sargent County, ND\"\t38081\n\"Roberts County, SD\"\t46109\t\"Day County, SD\"\t46037\n\"Roberts County, SD\"\t46109\t\"Grant County, SD\"\t46051\n\"Roberts County, SD\"\t46109\t\"Marshall County, SD\"\t46091\n\"Roberts County, SD\"\t46109\t\"Roberts County, SD\"\t46109\n\"Sanborn County, SD\"\t46111\t\"Aurora County, SD\"\t46003\n\"Sanborn County, SD\"\t46111\t\"Beadle County, SD\"\t46005\n\"Sanborn County, SD\"\t46111\t\"Davison County, SD\"\t46035\n\"Sanborn County, SD\"\t46111\t\"Hanson County, SD\"\t46061\n\"Sanborn County, SD\"\t46111\t\"Jerauld County, SD\"\t46073\n\"Sanborn County, SD\"\t46111\t\"Kingsbury County, SD\"\t46077\n\"Sanborn County, SD\"\t46111\t\"Miner County, SD\"\t46097\n\"Sanborn County, SD\"\t46111\t\"Sanborn County, SD\"\t46111\n\"Shannon County, SD\"\t46113\t\"Cherry County, NE\"\t31031\n\"Shannon County, SD\"\t46113\t\"Dawes County, NE\"\t31045\n\"Shannon County, SD\"\t46113\t\"Sheridan County, NE\"\t31161\n\"Shannon County, SD\"\t46113\t\"Bennett County, SD\"\t46007\n\"Shannon County, SD\"\t46113\t\"Custer County, SD\"\t46033\n\"Shannon County, SD\"\t46113\t\"Fall River County, SD\"\t46047\n\"Shannon County, SD\"\t46113\t\"Jackson County, SD\"\t46071\n\"Shannon County, SD\"\t46113\t\"Pennington County, SD\"\t46103\n\"Shannon County, SD\"\t46113\t\"Shannon County, SD\"\t46113\n\"Spink County, SD\"\t46115\t\"Beadle County, SD\"\t46005\n\"Spink County, SD\"\t46115\t\"Brown County, SD\"\t46013\n\"Spink County, SD\"\t46115\t\"Clark County, SD\"\t46025\n\"Spink County, SD\"\t46115\t\"Day County, SD\"\t46037\n\"Spink County, SD\"\t46115\t\"Faulk County, SD\"\t46049\n\"Spink County, SD\"\t46115\t\"Hand County, SD\"\t46059\n\"Spink County, SD\"\t46115\t\"Spink County, SD\"\t46115\n\"Stanley County, SD\"\t46117\t\"Dewey County, SD\"\t46041\n\"Stanley County, SD\"\t46117\t\"Haakon County, SD\"\t46055\n\"Stanley County, SD\"\t46117\t\"Hughes County, SD\"\t46065\n\"Stanley County, SD\"\t46117\t\"Jones County, SD\"\t46075\n\"Stanley County, SD\"\t46117\t\"Lyman County, SD\"\t46085\n\"Stanley County, SD\"\t46117\t\"Stanley County, SD\"\t46117\n\"Stanley County, SD\"\t46117\t\"Sully County, SD\"\t46119\n\"Stanley County, SD\"\t46117\t\"Ziebach County, SD\"\t46137\n\"Sully County, SD\"\t46119\t\"Dewey County, SD\"\t46041\n\"Sully County, SD\"\t46119\t\"Hughes County, SD\"\t46065\n\"Sully County, SD\"\t46119\t\"Hyde County, SD\"\t46069\n\"Sully County, SD\"\t46119\t\"Potter County, SD\"\t46107\n\"Sully County, SD\"\t46119\t\"Stanley County, SD\"\t46117\n\"Sully County, SD\"\t46119\t\"Sully County, SD\"\t46119\n\"Todd County, SD\"\t46121\t\"Cherry County, NE\"\t31031\n\"Todd County, SD\"\t46121\t\"Keya Paha County, NE\"\t31103\n\"Todd County, SD\"\t46121\t\"Bennett County, SD\"\t46007\n\"Todd County, SD\"\t46121\t\"Jackson County, SD\"\t46071\n\"Todd County, SD\"\t46121\t\"Mellette County, SD\"\t46095\n\"Todd County, SD\"\t46121\t\"Todd County, SD\"\t46121\n\"Todd County, SD\"\t46121\t\"Tripp County, SD\"\t46123\n\"Tripp County, SD\"\t46123\t\"Cherry County, NE\"\t31031\n\"Tripp County, SD\"\t46123\t\"Keya Paha County, NE\"\t31103\n\"Tripp County, SD\"\t46123\t\"Gregory County, SD\"\t46053\n\"Tripp County, SD\"\t46123\t\"Lyman County, SD\"\t46085\n\"Tripp County, SD\"\t46123\t\"Mellette County, SD\"\t46095\n\"Tripp County, SD\"\t46123\t\"Todd County, SD\"\t46121\n\"Tripp County, SD\"\t46123\t\"Tripp County, SD\"\t46123\n\"Turner County, SD\"\t46125\t\"Clay County, SD\"\t46027\n\"Turner County, SD\"\t46125\t\"Hutchinson County, SD\"\t46067\n\"Turner County, SD\"\t46125\t\"Lincoln County, SD\"\t46083\n\"Turner County, SD\"\t46125\t\"McCook County, SD\"\t46087\n\"Turner County, SD\"\t46125\t\"Minnehaha County, SD\"\t46099\n\"Turner County, SD\"\t46125\t\"Turner County, SD\"\t46125\n\"Turner County, SD\"\t46125\t\"Yankton County, SD\"\t46135\n\"Union County, SD\"\t46127\t\"Plymouth County, IA\"\t19149\n\"Union County,
